vi "Left-click Shortcut Menu.vi"() -> ()   [LabVIEW 2020]
doc: "This example shows how to display a context menu when you left-click a control. This example uses the Mouse Down? and Shortcut Menu Activation? filter events. In the Mouse Down? event, the example modifies the Button parameter so LabVIEW interprets a left-click as a right-click and fires the Shortcut Menu Activation? event."
panel:
  in  "Stop":bool
  in  "Left-click This Control":u16
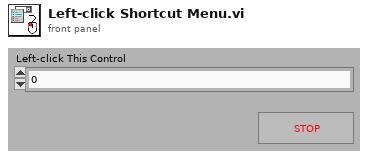
[diagram p1: front panel]
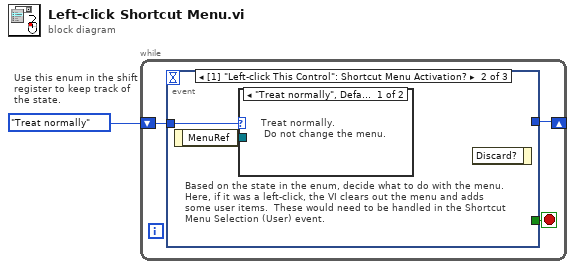
[diagram p0: block diagram]
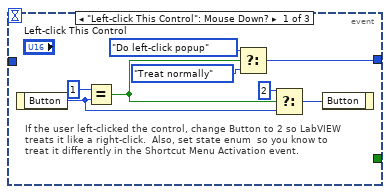
[diagram p2: hidden frame]
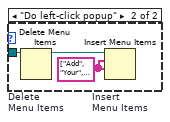
[diagram p3: hidden frame]
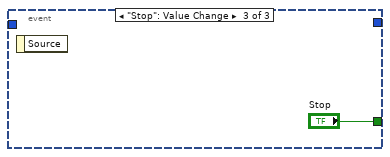
[diagram p4: hidden frame]
diagram:
  # "Use this enum in the shift \nregister to keep track of \nthe state."
  n1 = while {
    shift-right: [w3] -> _
    shift-left: enum16{"Treat normally", "Do left-click popup"}."Treat normally" ("Enum") -> [w2]
    stop <- w4 stop-if-true
    n2 = event shown="[1] \"Left-click This Control\": Shortcut Menu Activation?" {
      selector: _ -> [_ _ _]
      dyn-events: _ -> [_ _ _]
      timeout: _ -> [_ _ _]
      tunnel: [_ _ "Stop"] -> w4
      tunnel: [w12 _ _] -> w3
      tunnel: w2 -> [_ w14 _]
      event "Left-click This Control": Mouse Down? {
        # "If the user left-clicked the control, change Button to 2 so LabVIEW  treats it like a right-click.  Also, set state enum  so you know to treat it differently in the Shortcut Menu Activation event."
        n3 = event-data() -> ("Button"=w7:u16)  [unwired: 1 in]
        n4 = Equal?(x=u16 1, y=w7) -> (x = y?=w9:bool)
        n5 = Select(t=enum16{"Treat normally", "Do left-click popup"}."Do left-click popup" ("f"), s=w9, f=enum16{"Treat normally", "Do left-click popup"}."Treat normally" ("Enum")) -> (s? t:f=w12:enum16{"Treat normally", "Do left-click popup"})
        n6 = Select(t=u16 2, s=w9, f=w7) -> (s? t:f=w11:u16)
        n7 = event-data("Button"=w11) -> ()  [unwired: 1 in, 1 out]
      }
      event "Left-click This Control": Shortcut Menu Activation? {
        # "Based on the state in the enum, decide what to do with the menu.\nHere, if it was a left-click, the VI clears out the menu and adds\nsome user items.  These would need to be handled in the Shortcut\nMenu Selection (User) event."
        n8 = event-data() -> ("MenuRef"=w13:refnum<k9>)  [unwired: 1 in]
        n9 = case shown="\"Treat normally\", Default" w14 {
          tunnel: w13 -> [_ w17]
          frame "Treat normally", Default {
            # "Treat normally.\n Do not change the menu."
          }
          frame "Do left-click popup" {
            w15 = string[] ["Add", "Your", "Menu", "Items", "Here"]
            n10 = Delete Menu Items "Delete\nMenu Items"(9:w17) -> (3:w16:refnum<k9>)  [unwired: 3 in, 1 out]
            n11 = Insert Menu Items "Insert\nMenu Items"(7:w15, 8:w15, 9:w16) -> ()  [unwired: 3 in, 3 out]
          }
        }
        n12 = event-data() -> ()  [unwired: 2 in, 1 out]
      }
      event "Stop": Value Change {
        n13 = event-data() -> ()  [unwired: 1 in, 1 out]
      }
    }
  }
